vi "Main.vi"(8 "error in (no error)":errorcluster, 11 "TemplateBase in":refnum<class "PockelCell.lvclass">) -> (0 "error out":errorcluster, 3 "component":refnum<class "PockelCell.lvclass">)   [LabVIEW 2012, in "PockelCell.lvclass"]
doc: "Main VI of the component."
uses:
  PockelCell.lvclass
  Murmex/LabVIEW/Murmex/InitialiseMessage/InitialiseMessage.lvclass
  Murmex/LabVIEW/Murmex/TerminateMessage/TerminateMessage.lvclass
  <vilib>/Distrio/Murmex/Message/Message.lvclass
  Murmex/LabVIEW/Murmex/ConfigureMessage/ConfigureMessage.lvclass
  Murmex/LabVIEW/Murmex/StopMessage/StopMessage.lvclass
  Murmex/LabVIEW/Murmex/StartMessage/StartMessage.lvclass
  <vilib>/Distrio/Murmex/StartMessage/run mode enum.ctl
  <vilib>/Distrio/Murmex/StartMessage/StartMessage.lvclass
  Murmex/LabVIEW/Murmex/Murmex/update_cluster.ctl
  Murmex/LabVIEW/Murmex/Murmex/command_enum.ctl
  control/laser line PC.ctl
panel:
  in  "Tab Control":enum32{"Pockels Cell", "Debug"}(tab)
  in  "Duty cycle (%)":dbl(knob)=50.0 min=0.0 max=100.0 step=5.0 scale=0.0..100.0
  in  "Number of cycles":i32=1
  in  "Samples per cycle":i32=10
  in  "button:configure":bool
  in  "button:quit":bool
  in  "button::start inf":bool
  in  "button::start fin":bool
  in  "Analog Voltage":T1=3.0 items=["Empty", "445nm", "488nm", "515nm"]
  out "log":string
  in  "component ID":string
  in  "command":T2
  in  "button:send command":bool
  in  "generic command":string
  out "terminate?":bool
  # "digital out"
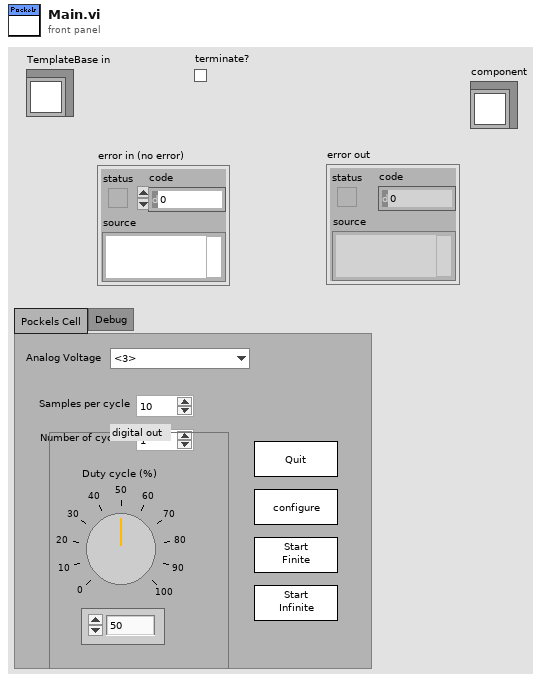
[diagram p1: front panel]
types:
  T1 = typedef "PockelCell.lvclass/laser line PC.ctl" = dbl
  T2 = typedef "Murmex.lvclass/command_enum.ctl" = enum16{"null", "initialise", "reset", "terminate", "acknowledge", "update", "inspect", "inform", "proceed", "start", "stop", "fetch", "configure", "generic"}
  T3 = typedef "Murmex.lvlib/StartMessage.lvclass/run mode enum.ctl" = enum16{"infinite", "finite"}
  T4 = enum8{"Enabled", "Disabled", "Disabled and Grayed Out"}
  T5 = typedef "Murmex.lvclass/update_cluster.ctl" = cluster{"target ID":string, "key chains":string[], "values":variant[]}
  T6 = typedef "Murmex.lvclass/Event type enumerations.ctl" = enum16{"before", "after"}
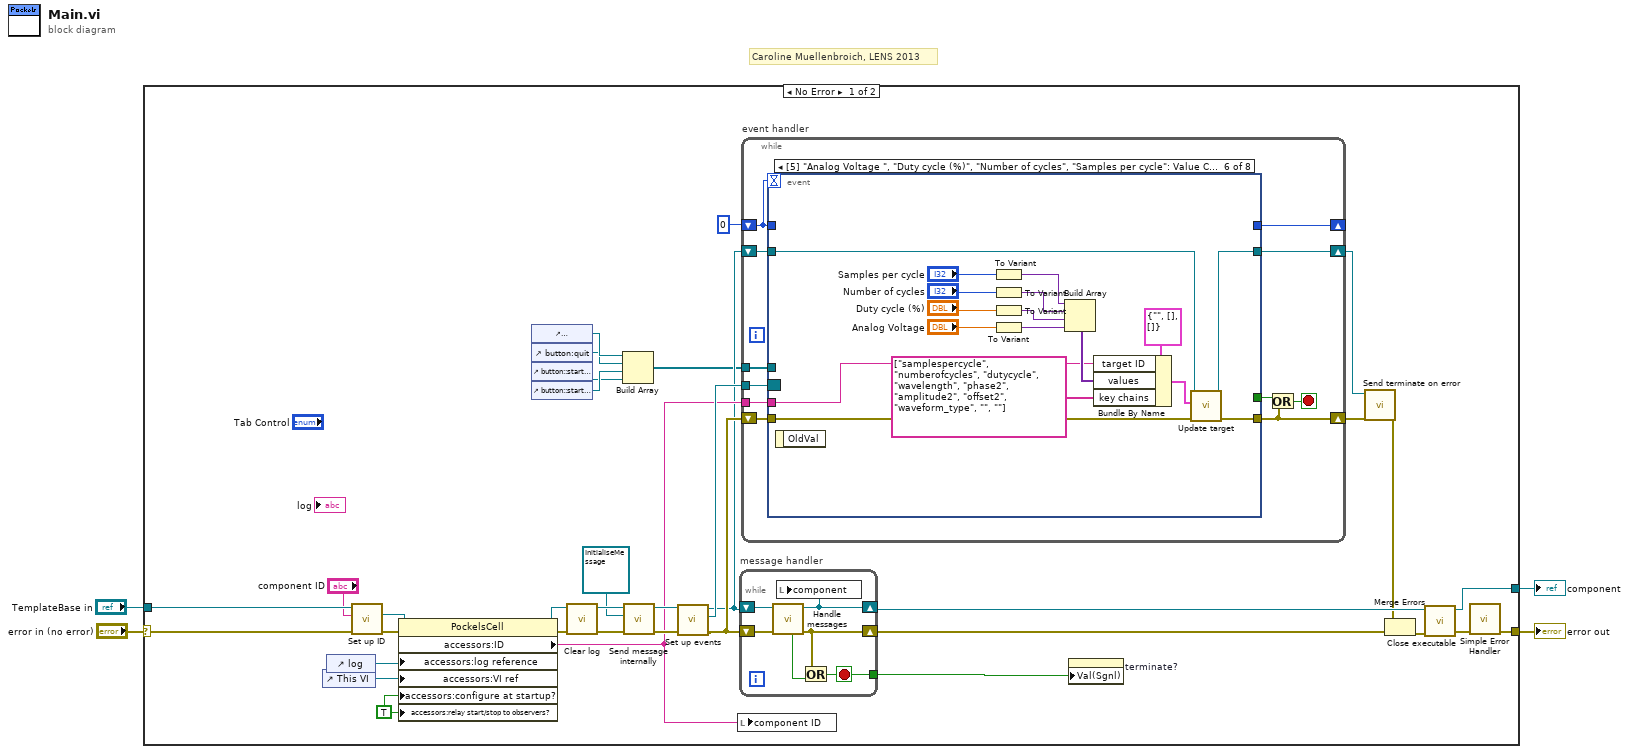
[diagram p0: block diagram]
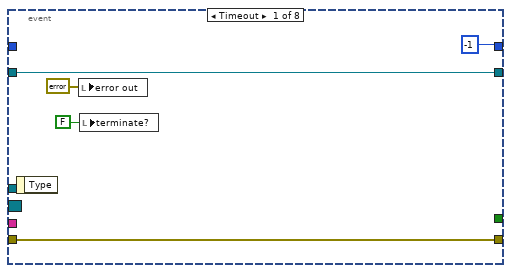
[diagram p2: hidden frame]
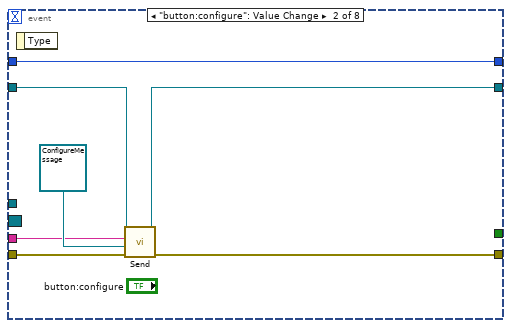
[diagram p3: hidden frame]
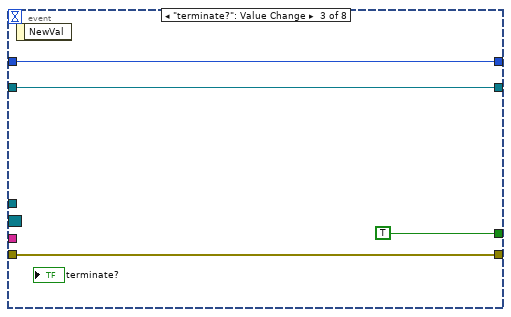
[diagram p4: hidden frame]
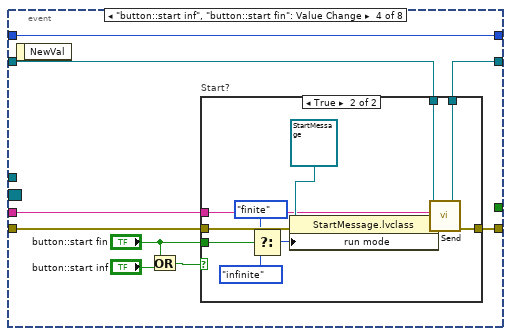
[diagram p5: hidden frame]
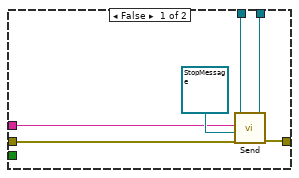
[diagram p6: hidden frame]
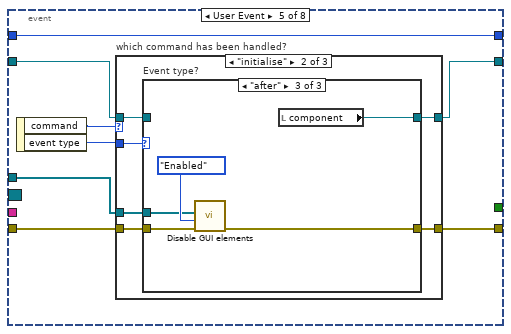
[diagram p7: hidden frame]
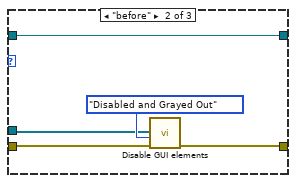
[diagram p10: hidden frame]
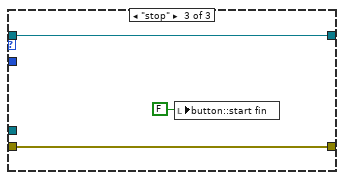
[diagram p11: hidden frame]
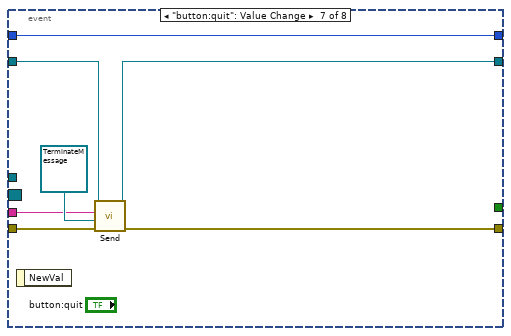
[diagram p12: hidden frame]
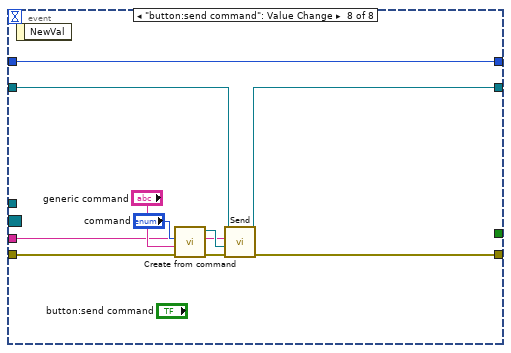
[diagram p13: hidden frame]
diagram:
  # "Caroline Muellenbroich, LENS 2013"
  n1 = case shown="No Error" "error in (no error)" {
    selector: "error in (no error)" -> [w26 w166]
    tunnel: [w15 w165] -> w4
    tunnel: "TemplateBase in" -> [w30 w165]
    tunnel: [w18 w166] -> w2
    frame No Error {
      w25 = TRUE ("configure at startup?")
      n2 = control-ref of="This VI"() -> (w37:refnum<vi>)
      n3 = control-ref of="log"() -> (w38:refnum<vi>)
      n4 = call "Set up ID.vi"("error in (no error)"=w26, "component ID"="component ID", "MurmexBase in"=w30) -> ("error out"=w31:errorcluster, "MurmexBase out"=w29:refnum<class "PockelCell.lvclass">)  [unwired: 6 in, 1 out]
      n5 = property class="PockelsCell"(reference=w29, error in=w31, "accessors:log reference"=w38, "accessors:VI ref"=w37, "accessors:configure at startup?"=w25, "accessors:relay start/stop to observers?"=w25) -> (reference out=w39:refnum<class "PockelCell.lvclass">, error out=w35:errorcluster, "accessors:ID"=w20:string)
      n6 = control-ref of="button:configure"() -> (w9:refnum<vi>)
      n7 = control-ref of="button:quit"() -> (w8:refnum<vi>)
      n8 = control-ref of="button::start inf"() -> (w6:refnum<vi>)
      n9 = control-ref of="button::start fin"() -> (w7:refnum<vi>)
      n10 = call "Clear log.vi"("error in (no error)"=w35, "MurmexBase in"=w39) -> ("error out"=w34:errorcluster, "MurmexBase out"=w36:refnum<class "PockelCell.lvclass">)  [unwired: 8 in]
      n11 = Build Array(w9, w8, w7, w6) -> (w5:refnum<vi>[])
      n12 = call "Send message internally.vi"("error in (no error)"=w34, "Message"=refnum<class "InitialiseMessage.lvclass"> refnum ("InitialiseMessage"), "Murmex in"=w36) -> ("error out"=w23:errorcluster, "Murmex out"=w24:refnum<class "PockelCell.lvclass">)  [unwired: 7 in]
      n13 = call "Set up events.vi"("error in (no error)"=w23, "MurmexBase in"=w24) -> ("error out"=w22:errorcluster, "Event Registration Refnum"=w21:refnum<event-registration>, "MurmexBase out"=w12:refnum<class "PockelCell.lvclass">)  [unwired: 7 in]
      n14 = local write "component ID"(w20) -> ()
      n15 = while "message handler" {
        shift-right: [w162] -> w27
        shift-left: w22 -> [w164]
        shift-right: [w159] -> w16
        shift-left: w12 -> [w163]
        tunnel: [w160] -> w32
        stop <- w160 stop-if-true
        n16 = call "Handle messages.vi"("error in (no error)"=w164, "Murmex in"=w163) -> ("error out"=w162:errorcluster, "Murmex out"=w159:refnum<class "PockelCell.lvclass">, "terminated?"=w161:bool)  [unwired: 7 in]
        n17 = local write "component"(w159) -> ()
        n18 = Or(x=w162, y=w161) -> (x .or. y?=w160:bool)
      }
      n19 = while "event handler" {
        shift-right: [w49] -> w13
        shift-left: w22 -> [w50]
        tunnel: w21 -> [w44]
        tunnel: w20 -> [w41]
        shift-right: [w46] -> _
        shift-left: 0 -> [w45]
        shift-right: [w42] -> w10
        shift-left: w12 -> [w43]
        tunnel: w5 -> [w40]
        stop <- w47 stop-if-true
        n20 = event shown="[5] \"Analog Voltage \", \"Duty cycle (%)\", \"Number of cycles\", \"Samples per cycle\": Value Change" {
          selector: w44 -> [_ _ _ _ _ _ _ _]
          dyn-events: _ -> [_ _ _ _ _ _ _ _]
          timeout: w45 -> [_ _ _ _ _ _ _ _]
          tunnel: w50 -> [w55 w60 w66 w74 w101 w135 w146 w158]
          tunnel: [w55 w59 w66 w73 w100 w132 w148 w156] -> w49
          tunnel: [_ _ TRUE _ _ _ _ _] -> w48
          tunnel: [-1 w62 w64 w67 w94 _ w142 w153] -> w46
          tunnel: w45 -> [_ w62 w64 w67 w94 _ w142 w153]
          tunnel: w43 -> [w51 w57 w63 w70 w97 w126 w144 w150]
          tunnel: [w51 w56 w63 w68 w95 w133 w143 w149] -> w42
          tunnel: w41 -> [_ w58 _ w69 _ w131 w145 w151]
          tunnel: w40 -> [_ _ _ _ w96 _ _ _]
          event Timeout {
            n21 = event-data() -> ()  [unwired: 1 in, 1 out]
            n22 = local write "error out"(errorcluster {"status"=FALSE, "code"=0, "source"=""} ("error out")) -> ()
            n23 = local write "terminate?"(FALSE ("terminate?")) -> ()
          }
          event "button:configure": Value Change {
            n24 = event-data() -> ()  [unwired: 1 in, 1 out]
            n25 = call "Send.vi"("error in (no error)"=w60, "Message"=refnum<class "ConfigureMessage.lvclass"> refnum ("ConfigureMessage"), "recipient"=w58, "Murmex in"=w57) -> ("error out"=w59:errorcluster, "Murmex out"=w56:refnum<class "PockelCell.lvclass">)  [unwired: 6 in]
          }
          event "terminate?": Value Change {
            n26 = event-data() -> ()  [unwired: 1 in, 1 out]
          }
          event "button::start inf", "button::start fin": Value Change {
            n27 = event-data() -> ()  [unwired: 1 in, 1 out]
            n28 = Or(x="button::start fin", y="button::start inf") -> (x .or. y?=w71:bool)
            n29 = case "Start?" shown="True" w71 {
              tunnel: w74 -> [w81 w92]
              tunnel: w69 -> [w76 w86]
              tunnel: w70 -> [w78 w89]
              tunnel: [w77 w88] -> w68
              tunnel: [w80 w87] -> w73
              tunnel: "button::start fin" -> [_ w82]
              frame False {
                n30 = call "Send.vi"("error in (no error)"=w81, "Message"=refnum<class "StopMessage.lvclass"> refnum ("StopMessage.lvclass"), "recipient"=w76, "Murmex in"=w78) -> ("error out"=w80:errorcluster, "Murmex out"=w77:refnum<class "PockelCell.lvclass">)  [unwired: 6 in]
              }
              frame True {
                n31 = Select(t=run_mode_enum."finite" ("run mode"), s=w82, f=run_mode_enum."infinite" ("run mode")) -> (s? t:f=w83:T3)
                n32 = property class="StartMessage.lvclass"(reference=refnum<class "StartMessage.lvclass"> refnum ("StartMessage"), error in=w92, "run mode"=w83) -> (reference out=w90:refnum<class "StartMessage.lvclass">, error out=w91:errorcluster)
                n33 = call "Send.vi"("error in (no error)"=w91, "Message"=w90, "recipient"=w86, "Murmex in"=w89) -> ("error out"=w87:errorcluster, "Murmex out"=w88:refnum<class "PockelCell.lvclass">)  [unwired: 6 in]
              }
            }
          }
          event User Event {
            n34 = event-data() -> ("command"=w99:T2, "event type"=w98:T6)  [unwired: 1 in]
            n35 = case "which command has been handled?" shown="\"initialise\"" w99 {
              tunnel: w98 -> [_ w109 _]
              tunnel: w101 -> [w103 w108 w122]
              tunnel: [w103 w107 w122] -> w100
              tunnel: [w102 w106 w124] -> w95
              tunnel: w97 -> [w102 w105 w124]
              tunnel: w96 -> [_ w104 _]
              frame Default {
              }
              frame "initialise" {
                n36 = case "Event type?" shown="\"after\"" w109 {
                  tunnel: w108 -> [w110 w114 w120]
                  tunnel: [w110 w113 w117] -> w107
                  tunnel: [w111 w116 w121] -> w106
                  tunnel: w105 -> [w111 w116 _]
                  tunnel: w104 -> [_ w112 w118]
                  frame Default {
                  }
                  frame "before" {
                    n37 = call "Disable GUI elements.vi"("error in (no error)"=w114, "enabled state"=T4."Disabled and Grayed Out" ("Disabled"), "control refs"=w112) -> ("error out"=w113:errorcluster)  [unwired: 8 in]
                  }
                  frame "after" {
                    n38 = call "Disable GUI elements.vi"("error in (no error)"=w120, "enabled state"=T4."Enabled", "control refs"=w118) -> ("error out"=w117:errorcluster)  [unwired: 8 in]
                    n39 = local read "component"() -> (w121:refnum<class "PockelCell.lvclass">)
                  }
                }
              }
              frame "stop" {
                n40 = local write "button::start fin"(FALSE ("button::start")) -> ()
              }
            }
          }
          event "Duty cycle (%)", "Number of cycles", "Samples per cycle": Value Change {
            n41 = event-data() -> ()  [unwired: 1 in, 1 out]
            n42 = To Variant(anything="Samples per cycle") -> (Variant=w130:variant)
            n43 = To Variant(anything="Number of cycles") -> (Variant=w141:variant)
            n44 = To Variant(anything="Duty cycle (%)") -> (Variant=w140:variant)
            n45 = To Variant(anything="Analog Voltage") -> (Variant=w139:variant)
            n46 = Build Array(w130, w141, w140, w139) -> (w138:variant[])
            n47 = Bundle By Name(cluster=T5 {"target ID"="", "key chains"=[], "values"=[]} ("update cluster"), "target ID"=w131, "values"=w138, "key chains"=string[] ["samplespercycle", "numberofcycles", "dutycycle", "wavelength", "phase2", "amplitude2", "offset2", "waveform_type", "", ""]) -> (w134:T5)
            n48 = call "Update target.vi"("error in (no error)"=w135, "update cluster"=w134, "MurmexBase in"=w126) -> ("error out"=w132:errorcluster, "MurmexBase out"=w133:refnum<class "PockelCell.lvclass">)  [unwired: 7 in]
          }
          event "button:quit": Value Change {
            n49 = event-data() -> ()  [unwired: 1 in, 1 out]
            n50 = call "Send.vi"("error in (no error)"=w146, "Message"=refnum<class "TerminateMessage.lvclass"> refnum ("TerminateMessage"), "recipient"=w145, "Murmex in"=w144) -> ("error out"=w148:errorcluster, "Murmex out"=w143:refnum<class "PockelCell.lvclass">)  [unwired: 6 in]
          }
          event "button:send command": Value Change {
            n51 = event-data() -> ()  [unwired: 1 in, 1 out]
            n52 = call <vilib>:"Create from command.vi"("error in (no error)"=w158, "generic command"="generic command", "command"="command") -> ("error out"=w152:errorcluster, "Message out"=w157:refnum<class "Message.lvclass">)  [unwired: 7 in]
            n53 = call "Send.vi"("error in (no error)"=w152, "Message"=w157, "recipient"=w151, "Murmex in"=w150) -> ("error out"=w156:errorcluster, "Murmex out"=w149:refnum<class "PockelCell.lvclass">)  [unwired: 6 in]
          }
        }
        n54 = Or(x=w48, y=w49) -> (x .or. y?=w47:bool)
      }
      n55 = property on="terminate?" class="Bool (strict)"("Val(Sgnl)"=w32) -> ()  [unwired: 2 in, 2 out]
      n56 = call "Send terminate on error.vi"("error in (no error)"=w13, "Murmex in"=w10) -> ("error out"=w14:errorcluster)  [unwired: 8 in, 1 out]
      n57 = Merge Errors(w14, w27) -> (w17:errorcluster)
      n58 = call "Close executable.vi"("error in (no error)"=w17, "MurmexBase in"=w16) -> ("error out"=w19:errorcluster, "MurmexBase out"=w15:refnum<class "PockelCell.lvclass">)  [unwired: 8 in]
      n59 = call <vilib>:"Simple Error Handler.vi"("error in (no error)"=w19) -> ("error out"=w18:errorcluster)  [unwired: 4 in, 4 out]
    }
    frame Error {
    }
  }
  "error out" <- w2
  "component" <- w4
